vi "Set Timing.vi"(8 "error in (no error)":errorcluster, 10 "Target Time":dbl format="%.2f", 11 "Car Wash Controller in":refnum<class "Car Wash Controller.lvclass">) -> (0 "error out":errorcluster, 3 "Car Wash Controller out":refnum<class "Car Wash Controller.lvclass">)   [LabVIEW 2019, in "Car Wash Controller.lvlib" / "Car Wash Controller.lvclass"]
uses:
  Car Wash Controller.lvclass
  Car Wash Controller.lvclass/Car Wash Controller.ctl
  Sim Wash Display Console/Sim Wash Display Console Messages/Write Remaining timing Msg/Write Remaining timing Msg.lvclass/Write Remaining timing Msg.ctl
  <vilib>/ActorFramework/Message Enqueuer/Message Enqueuer.lvclass/Message Enqueuer.ctl
  <vilib>/ActorFramework/Message Enqueuer/Enqueue.vi
  Sim Wash Display Console/Sim Wash Display Console Messages/Write Remaining timing Msg/Write Remaining timing Msg.lvclass
  C:/Program Files (x86)/National Instruments/LabVIEW 2019/vi.lib/ActorFramework/Message/Message.lvclass
  <vilib>/ActorFramework/Message Priority Queue/Priority Enqueue.vi
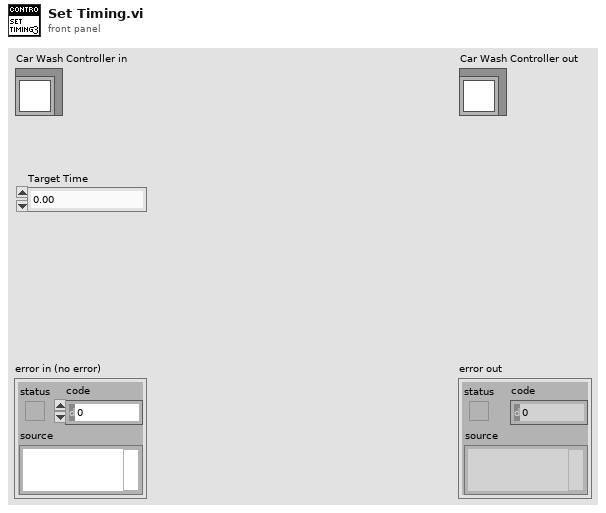
[diagram p1: front panel]
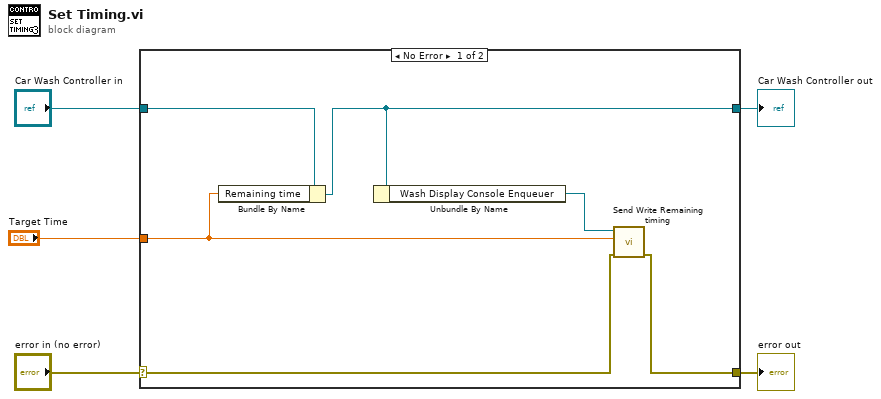
[diagram p0: block diagram]
diagram:
  n1 = case shown="No Error" "error in (no error)" {
    selector: "error in (no error)" -> [w10 w13]
    tunnel: [w9 w13] -> w4
    tunnel: [w6 w12] -> w2
    tunnel: "Car Wash Controller in" -> [w8 w12]
    tunnel: "Target Time" -> [w7 _]
    frame No Error {
      n2 = Bundle By Name(cluster=w8, "Remaining time"=w7) -> (w6:refnum<class "Car Wash Controller.lvclass">)
      n3 = Unbundle By Name(w6) -> ("Wash Display Console Enqueuer"=w11:refnum<class "Message Enqueuer.lvclass">)
      n4 = call "Send Write Remaining timing.vi"("error in (no error)"=w10, "Timing Remaining"=w7, "Message Enqueuer"=w11) -> ("error out"=w9:errorcluster)  [unwired: 7 in, 1 out]
    }
    frame Error {
    }
  }
  "error out" <- w4
  "Car Wash Controller out" <- w2
